vi "Read Waveform Osciloscope.vi"(8 "error in (no error)":errorcluster, 10 "ReadWaveform":T1={"TEKTRONIX READ-WAVEFORM 2"={"Source (0: Channel 1)"=0, "Timeout (10000 ms) 2"=10000}, "EDU-X-1200A- READ-WAVEFORM"={"Bind Source Channel (2: None)"=2, "Timeout (10000 ms)"=10000, "Source Channel (0: Channel 1)"=0}} {"EDU-X-1200A- READ-WAVEFORM"."Source Channel (0: Channel 1)" items=["Channel 1"=0, "Channel 2"=1, "Channel 3"=2, "Channel 4"=3, "Waveform Memory 1"=5, "Waveform Memory 2"=6, "Serial Bus 1"=7, "Serial Bus 2"=8, "Digital Bus Low"=9, "Digital Bus High "=10, "Digital Bus 1"=11, "Digital Bus 2"=12, "External"=29, "Function 1"=32, "Function 2"=33, "Function 3"=34, "Function 4"=35, "Math 1"=36, "Math 2"=37, "Math 3"=38, "Math 4"=39, "FFT"=40, "Analog Bus"=41]; "EDU-X-1200A- READ-WAVEFORM"."Bind Source Channel (2: None)" items=["Sub Source 0", "Sub Source 1", "None"]; "TEKTRONIX READ-WAVEFORM 2"."Source (0: Channel 1)" items=["Channel 1", "Channel 2", "Channel 3", "Channel 4", "Math", "Reference A", "Reference B", "Reference C", "Reference D", "FFT"]}, 11 "OsciloscopeClass in":refnum<class "OsciloscopeClass.lvclass">) -> (0 "error out":errorcluster, 2 "Waveform Data":waveform(dbl)(graph), 3 "OsciloscopeClass out":refnum<class "OsciloscopeClass.lvclass">)   [LabVIEW 2020, in "OsciloscopeClass.lvclass"]
uses:
  OsciloscopeClass.lvclass
  TypeDefs/ReadWaveform--cluster.ctl
  <vilib>/measure/NI_MABase.lvlib
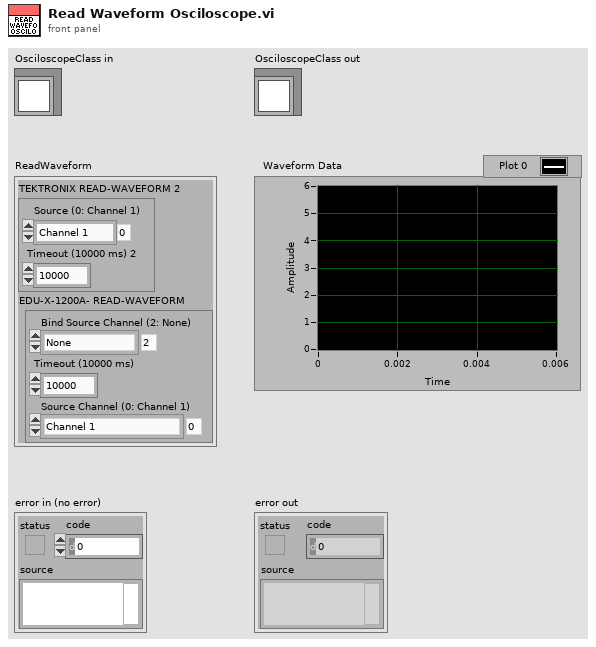
[diagram p1: front panel]
types:
  T1 = typedef "ReadWaveform--cluster.ctl" = cluster{"TEKTRONIX READ-WAVEFORM 2":cluster{"Source (0: Channel 1)":u16, "Timeout (10000 ms) 2":u32}, "EDU-X-1200A- READ-WAVEFORM":cluster{"Bind Source Channel (2: None)":i32, "Timeout (10000 ms)":u32, "Source Channel (0: Channel 1)":i32}}
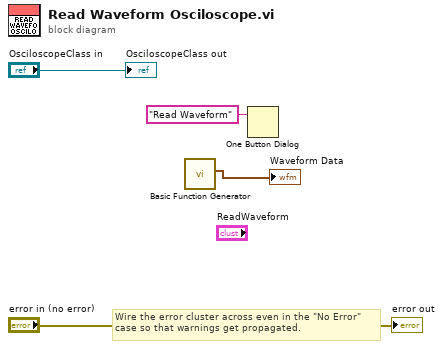
[diagram p0: block diagram]
diagram:
  # "Wire the error cluster across even in the \"No Error\"\ncase so that warnings get propagated."
  n1 = call <vilib>:"Basic Function Generator.vi"() -> ("signal out"=→"Waveform Data":waveform(dbl))  [unwired: 9 in, 2 out]
  n2 = One Button Dialog(message="Read Waveform") -> ()  [unwired: 1 in, 1 out]
  "error out" <- "error in (no error)"
  "OsciloscopeClass out" <- "OsciloscopeClass in"
